vi "Server_OPC_UA.vi"() -> ()   [LabVIEW 2025]
uses:
  <vilib>/OPCUA/controls/NodeId.ctl
  <vilib>/OPCUA/controls/Data Type.ctl
  <vilib>/OPCUA/server/Create2.vi
  <vilib>/OPCUA/NI OPC UA Server.lvlib
panel:
  in  "Stop":bool
  out "item node ID":T1
  out "server endpoint URL":string
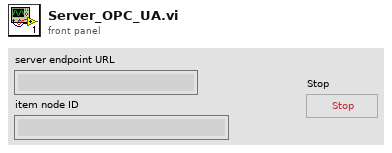
[diagram p1: front panel]
types:
  T1 = typedef "NodeId.ctl" = string
  T2 = typedef "Data Type.ctl" = u16
  T3 = cluster{"name":string, "data type":T2, "access level":u16, "description":string}
  T4 = typedef "OPC UA Server Refnum.ctl" = refnum<k21>
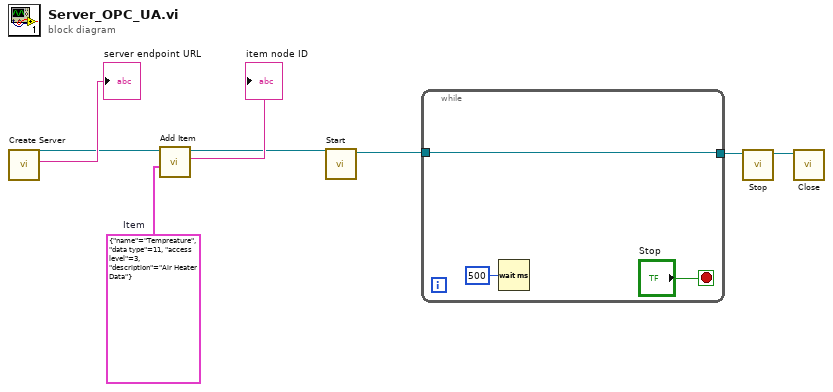
[diagram p0: block diagram]
diagram:
  w1 = T3 {"name"="Tempreature", "data type"=11, "access level"=3, "description"="Air Heater Data"}  # Item
  n1 = call-poly <vilib>:"Create Server.vi"() -> ("server endpoint URL"=→"server endpoint URL":string, "OPC UA server refnum out"=w6:T4)  [unwired: 9 in, 1 out]
  n2 = call <vilib>:"Add Item.vi"("item"=w1, "OPC UA server refnum in"=w6) -> ("item node ID"=→"item node ID":T1, "OPC UA server refnum out"=w5:T4)  [unwired: 5 in, 2 out]
  n3 = call <vilib>:"Start.vi"("OPC UA server refnum in"=w5) -> ("OPC UA server refnum out"=w4:T4)  [unwired: 8 in, 2 out]
  n4 = while {
    tunnel: w4 -> [w9]
    tunnel: [w9] -> w3
    stop <- "Stop" stop-if-true
    n5 = Wait (ms)(milliseconds to wait=u32 500) -> ()  [unwired: 1 out]
  }
  n6 = call <vilib>:"Stop.vi"("OPC UA server refnum in"=w3) -> ("OPC UA server refnum out"=w2:T4)  [unwired: 9 in, 1 out]
  n7 = call <vilib>:"Close.vi"("OPC UA server refnum in"=w2) -> ()  [unwired: 10 in, 1 out]
